vi "lockin - Restore Saved AO.vi"(8 "error in (no error)":errorcluster, 11 "Lockin.DAQ":refnum<class "Lockin.DAQ.lvclass">) -> (0 "error out":errorcluster, 3 "Lockin.DAQ out":refnum<class "Lockin.DAQ.lvclass">)   [LabVIEW 2019, in "Lockin.DAQ.lvclass"]
uses:
  Lockin.DAQ.lvclass
  Lockin.DAQ.lvclass/Lockin.DAQ.ctl
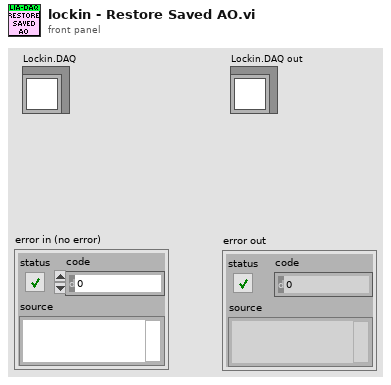
[diagram p1: front panel]
types:
  T1 = typedef "Lockin.DAQ.lvclass/AO-cluster.ctl" = T2[]
  T2 = typedef "Instrument.Lockin.UI.lvclass/AO Channel--Cluster.ctl" = cluster{"Enable?":bool, "Channel":i32, "Amplitude":dbl, "Offset":dbl, "Frequency":dbl, "Phase":dbl, "Function":T3, "Sweeping?":bool}
  T3 = typedef "Lockin.DAQ.lvclass/Function-enum.ctl" = enum16{"Sine", "Triangle", "Square"}
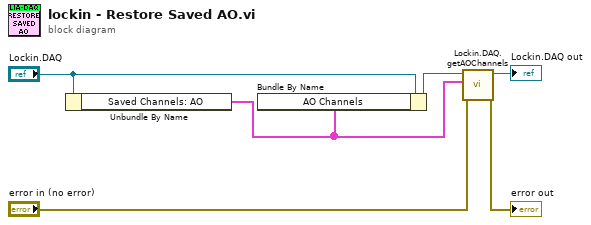
[diagram p0: block diagram]
diagram:
  n1 = Unbundle By Name("Lockin.DAQ") -> ("Saved Channels: AO"=w2:T1)
  n2 = Bundle By Name(cluster="Lockin.DAQ", "AO Channels"=w2) -> (w3:refnum<class "Lockin.DAQ.lvclass">)
  n3 = call "Lockin.DAQ.getAOChannels.vi"("error in (no error)"="error in (no error)", "Channels: AO"=w2, "Lockin.DAQ"=w3) -> ("error out"=→"error out":errorcluster, "Lockin.DAQ"=→"Lockin.DAQ out":refnum<class "Lockin.DAQ.lvclass">)  [unwired: 7 in]
